vi "Data_get.vi"() -> ()   [LabVIEW 2009]
uses:
  <vilib>/Analysis/2dsp.llb/Real FFT.vi
  <vilib>/Analysis/NI_AALPro.lvlib
panel:
  in  "Repetition rate (Hz)":ext=2.5
  in  "Chirp start (MHz)":ext=2.5
  in  "Filter up to (MHz)":ext=2.5
  in  "Amount of averagings":u32
  out "Data":dbl[](array[numeric])
  out "XY Graph 5":cluster{ext[], dbl[]}(graph)
  out "FFT (Im)":dbl[](array[numeric])
  out "FFT (Re)":dbl[](array[numeric])
  out "Final array":ext[][](array[numeric])
  out "size(s)":i32
  in  "ns/div":u32
  in  "ps/point":u32
  out "Oscilloscope Data":dbl[](array[numeric])
  in  "Channel Number":u16=1
  out "Oscilloscope graph":dbl[](graph)
  in  "Stop":bool
  in  "TDS VISA Port":refnum<visa-resource-name>="GPIB0::1::INSTR"
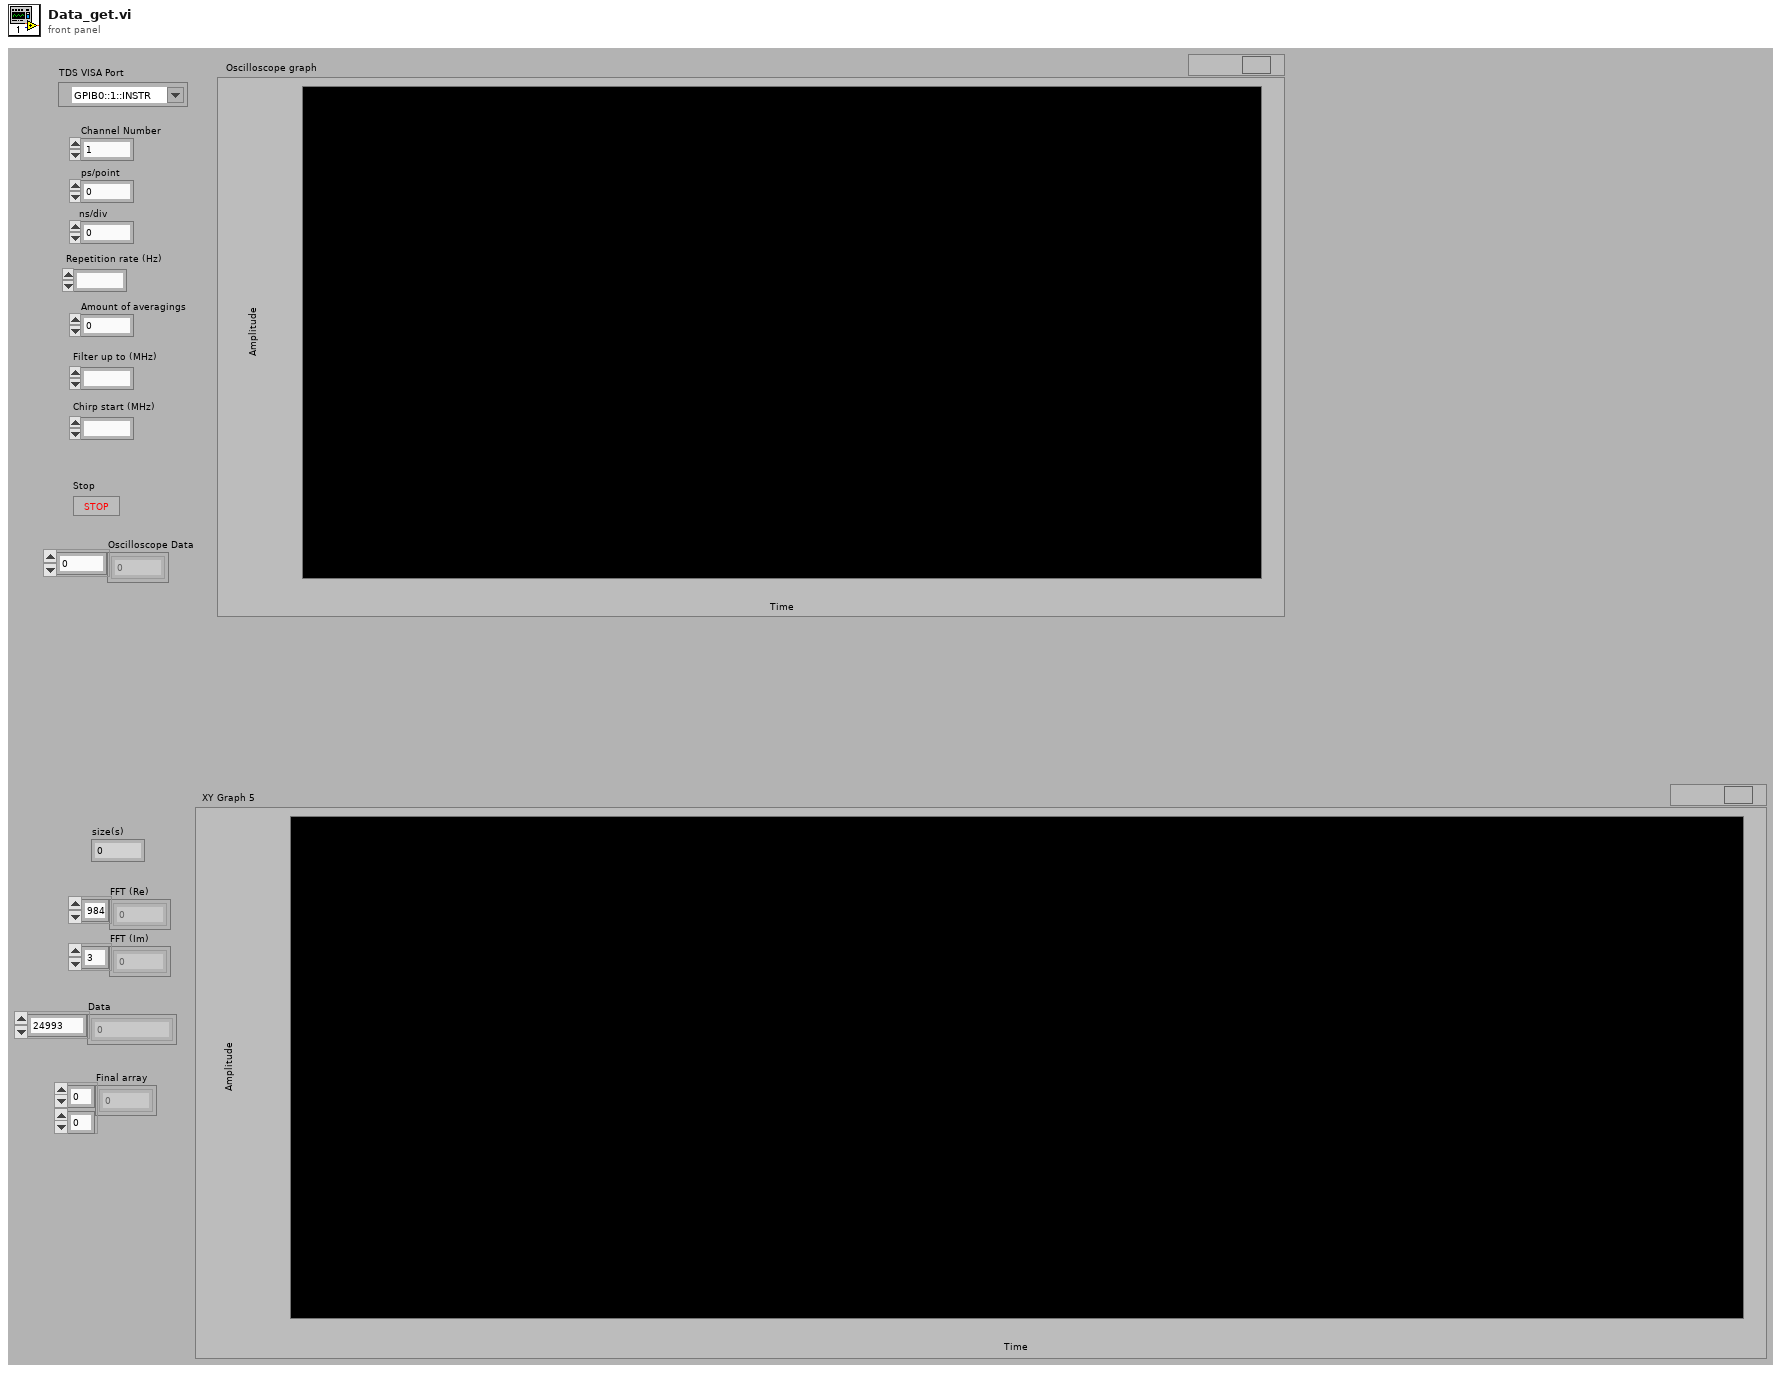
[diagram p1: front panel]
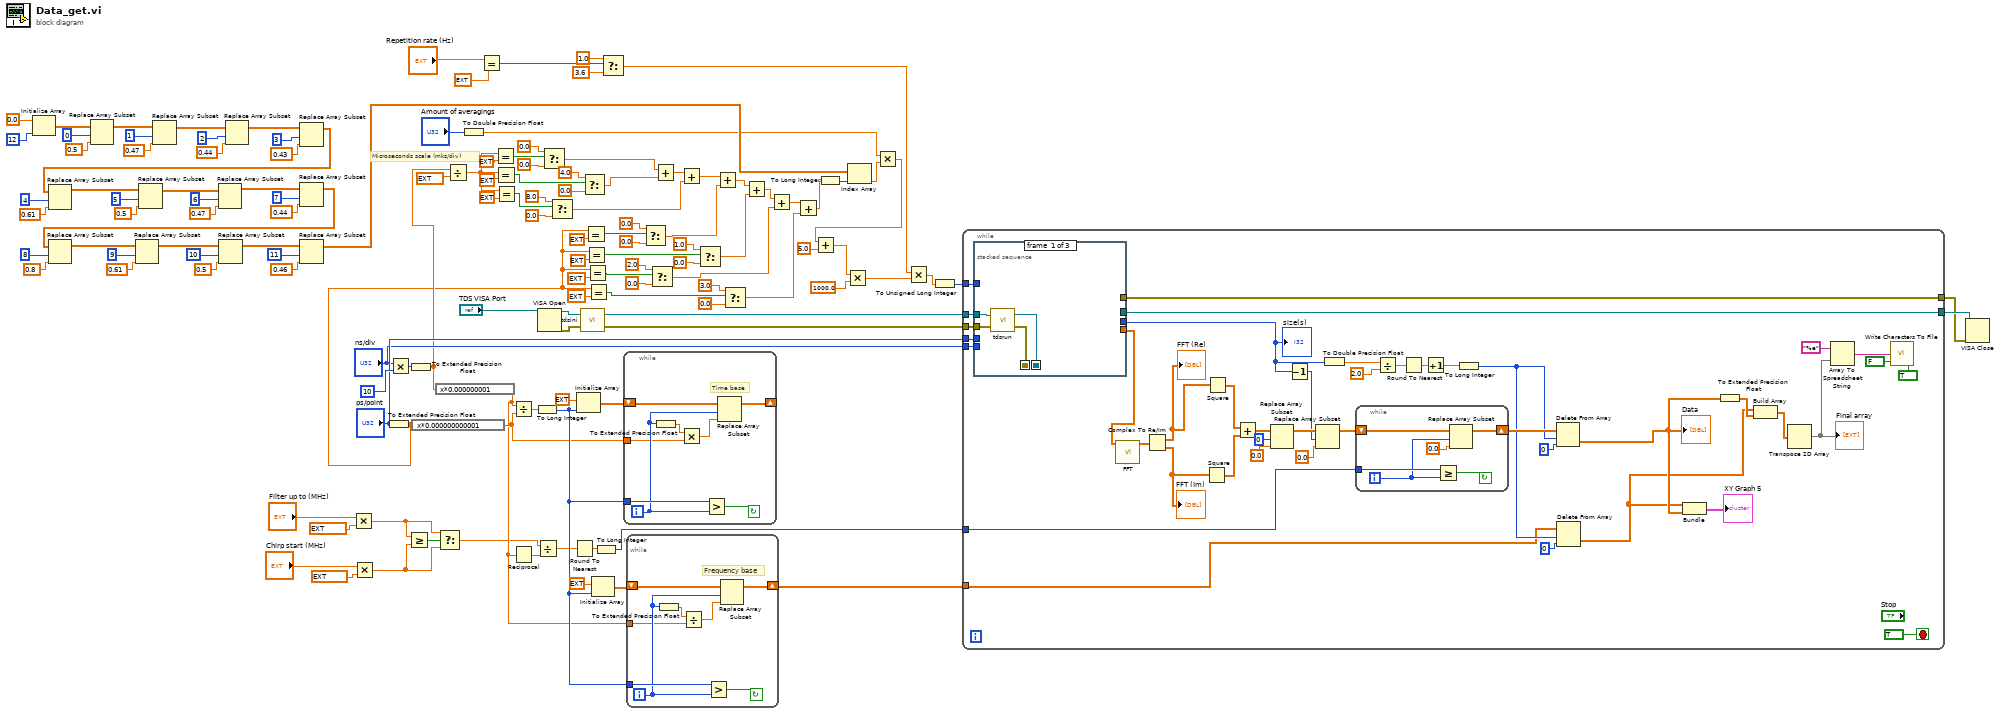
[diagram p0: block diagram]
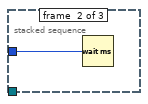
[diagram p2: hidden frame]
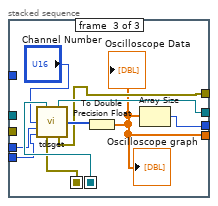
[diagram p3: hidden frame]
diagram:
  # "Microseconds scale (mks/div)"
  n1 = Initialize Array(0.0 ("element"), 12 ("dimension size")) -> (w109:dbl[])
  n2 = Replace Array Subset(array=w109, new element=0.5 ("new element/subarray"), index=0) -> (w104:dbl[])
  n3 = Replace Array Subset(array=w104, new element=0.47 ("new element/subarray"), index=1) -> (w83:dbl[])
  n4 = Replace Array Subset(array=w83, new element=0.44 ("new element/subarray"), index=2) -> (w82:dbl[])
  n5 = Replace Array Subset(array=w82, new element=0.43 ("new element/subarray"), index=3) -> (w81:dbl[])
  n6 = Replace Array Subset(array=w81, new element=0.61 ("new element/subarray"), index=4) -> (w80:dbl[])
  n7 = Replace Array Subset(array=w80, new element=0.5 ("new element/subarray"), index=5) -> (w79:dbl[])
  n8 = Replace Array Subset(array=w79, new element=0.47 ("new element/subarray"), index=6) -> (w78:dbl[])
  n9 = Replace Array Subset(array=w78, new element=0.44 ("new element/subarray"), index=7) -> (w77:dbl[])
  n10 = Replace Array Subset(array=w77, new element=0.8 ("new element/subarray"), index=8) -> (w76:dbl[])
  n11 = Replace Array Subset(array=w76, new element=0.61 ("new element/subarray"), index=9) -> (w75:dbl[])
  n12 = Replace Array Subset(array=w75, new element=0.5 ("new element/subarray"), index=10) -> (w74:dbl[])
  n13 = Replace Array Subset(array=w74, new element=0.46 ("new element/subarray"), index=11) -> (w32:dbl[])
  n14 = Multiply(x="Filter up to (MHz)", y=ext 1000000.0) -> (x*y=w12:ext)
  n15 = Multiply(x="Chirp start (MHz)", y=ext 1000000.0) -> (x*y=w9:ext)
  n16 = To Extended Precision Float(1:"ps/point") -> (0:w25:ext)
  n17 = Multiply(x="ns/div", y=u32 10) -> (x*y=w125:u32)
  n18 = Greater Or Equal?(x=w12, y=w9) -> (x >= y?=w21:bool)
  n19 = To Extended Precision Float(1:w125) -> (0:w113:ext)
  n20 = expression code="x*0.000000000001"(w25) -> (w114:ext)
  n21 = expression code="x*0.000000001"(w113) -> (w20:ext)
  n22 = Select(t=w12, s=w21, f=w9) -> (s? t:f=w18:ext)
  n23 = Divide(x=w113, y=ext 10000.0) -> (x/y=w73:ext)
  n24 = To Double Precision Float(number="Amount of averagings") -> (double precision float=w28:dbl)
  n25 = Equal?(x="Repetition rate (Hz)", y=ext 2.5) -> (x = y?=w7:bool)
  n26 = Equal?(x=w73, y=ext 1.0) -> (x = y?=w65:bool)
  n27 = Equal?(x=w73, y=ext 2.0) -> (x = y?=w60:bool)
  n28 = Equal?(x=w73, y=ext 4.0) -> (x = y?=w57:bool)
  n29 = Divide(x=w20, y=w114) -> (x/y=w124:ext)
  n30 = Reciprocal(x=w20) -> (1/x=w19:ext)
  n31 = To Long Integer(number=w124) -> (32bit integer=w116:i32)
  n32 = Divide(x=w18, y=w19) -> (x/y=w17:ext)
  n33 = VISA Open(VISA resource name="TDS VISA Port") -> (VISA resource name=w130:refnum<visa-resource-name>, error out=w131:errorcluster)  [unwired: 4 in]
  n34 = Select(t=0.0, s=w65, f=0.0) -> (s? t:f=w44:dbl)
  n35 = Select(t=8.0, s=w57, f=0.0) -> (s? t:f=w41:dbl)
  n36 = Round To Nearest(number=w17) -> (nearest integer value=w16:ext)
  n37 = Initialize Array(ext 0.0 ("element"), w116) -> (w120:ext[])
  n38 = call "tdsini.vi"("Error In (No Error)"=w131, "VISA Port In"=w130) -> ("Error Out"=w132:errorcluster, "VISA Port Out"=w133:refnum<visa-resource-name>)
  n39 = Select(t=4.0, s=w60, f=0.0) -> (s? t:f=w43:dbl)
  n40 = Equal?(x=w25, y=ext 25.0) -> (x = y?=w48:bool)
  n41 = Equal?(x=w25, y=ext 50.0) -> (x = y?=w47:bool)
  n42 = Equal?(x=w25, y=ext 100.0) -> (x = y?=w46:bool)
  n43 = Equal?(x=w25, y=ext 200.0) -> (x = y?=w45:bool)
  n44 = Initialize Array(ext 0.0 ("element"), w116) -> (w118:ext[])
  n45 = To Long Integer(number=w16) -> (32bit integer=w15:i32)
  n46 = Select(t=1.0, s=w7, f=3.6) -> (s? t:f=w4:dbl)
  n47 = while {
    tunnel: w116 -> [w140]
    shift-right: [w138] -> _
    shift-left: w120 -> [w139]
    tunnel: w114 -> [w135]
    i -> [w137]
    stop <- w141 continue-if-true
    # "Time base"
    n48 = To Extended Precision Float(1:w137) -> (0:w136:ext)
    n49 = Multiply(x=w136, y=w135) -> (x*y=w134:ext)
    n50 = Greater?(x=w140, y=w137) -> (0:w141:bool)
    n51 = Replace Array Subset(array=w139, new element=w134, index=w137) -> (w138:ext[])
  }
  n52 = while {
    tunnel: w116 -> [w148]
    shift-right: [w146] -> w117
    shift-left: w118 -> [w147]
    tunnel: w20 -> [w143]
    i -> [w145]
    stop <- w149 continue-if-true
    # "Frequency base"
    n53 = To Extended Precision Float(1:w145) -> (0:w144:ext)
    n54 = Divide(x=w144, y=w143) -> (x/y=w142:ext)
    n55 = Greater?(x=w148, y=w145) -> (0:w149:bool)
    n56 = Replace Array Subset(array=w147, new element=w142, index=w145) -> (w146:ext[])
  }
  n57 = Select(t=0.0, s=w48, f=0.0) -> (s? t:f=w39:dbl)
  n58 = Select(t=2.0, s=w46, f=0.0) -> (s? t:f=w35:dbl)
  n59 = Add(x=w44, y=w43) -> (x+y=w42:dbl)
  n60 = Add(x=w42, y=w41) -> (x+y=w40:dbl)
  n61 = Select(t=1.0, s=w47, f=0.0) -> (s? t:f=w37:dbl)
  n62 = Add(x=w40, y=w39) -> (x+y=w38:dbl)
  n63 = Select(t=3.0, s=w45, f=0.0) -> (s? t:f=w33:dbl)
  n64 = Add(x=w38, y=w37) -> (x+y=w36:dbl)
  n65 = Add(x=w36, y=w35) -> (x+y=w34:dbl)
  n66 = Add(x=w34, y=w33) -> (x+y=w30:dbl)
  n67 = To Long Integer(number=w30) -> (32bit integer=w31:i32)
  n68 = Index Array(array=w32, index=w31) -> (element=w29:dbl)
  n69 = Multiply(x=w28, y=w29) -> (x*y=w24:dbl)
  n70 = Add(x=w24, y=5.0) -> (x+y=w22:dbl)
  n71 = Multiply(x=w22, y=1000.0) -> (x*y=w3:dbl)
  n72 = Multiply(x=w4, y=w3) -> (x*y=w2:dbl)
  n73 = To Unsigned Long Integer(number=w2) -> (unsigned 32bit integer=w26:u32)
  n74 = while {
    tunnel: [w189] -> w127
    tunnel: [w190] -> w128
    tunnel: w132 -> [w191]
    tunnel: w133 -> [w192]
    tunnel: "ps/point" -> [w188]
    tunnel: "ns/div" -> [w187]
    tunnel: w117 -> [w151]
    tunnel: w26 -> [w168]
    tunnel: w15 -> [w164]
    stop <- TRUE stop-if-true
    n75 = stacked-sequence {
      seq-local: [w200 _ _] -> [_ _ w213]
      seq-local: [w199 _ _] -> [_ _ w206]
      tunnel: w192 -> [w201 _ _]
      tunnel: w191 -> [w202 _ _]
      tunnel: [_ _ w211] -> w190
      tunnel: [_ _ w210] -> w189
      tunnel: w188 -> [_ _ w208]
      tunnel: w187 -> [_ _ w207]
      tunnel: [_ _ w205] -> w162
      tunnel: [_ _ w204] -> w180
      tunnel: w168 -> [_ w203 _]
      frame #0 {
        n76 = call "tdsrun.vi"("Error In (No Error)"=w202, "VISA Port In"=w201) -> ("Error Out"=w199:errorcluster, "VISA Port Out"=w200:refnum<visa-resource-name>)
      }
      frame #1 {
        n77 = Wait (ms)(milliseconds to wait=w203) -> ()  [unwired: 1 out]
      }
      frame #2 {
        n78 = call "tdsget.vi"("VISA Port In"=w213, "Channel Number"="Channel Number", "ps/point"=w208, "ns/div"=w207, "Error In (No Error)"=w206) -> ("VISA Port Out"=w211:refnum<visa-resource-name>, "TDS Data"=w212:u16[], "Error Out"=w210:errorcluster)  [unwired: 8 in]
        n79 = To Double Precision Float(number=w212) -> (double precision float=w204:dbl[])
        "Oscilloscope graph" <- w204
        "Oscilloscope Data" <- w204
        n80 = Array Size(array=w204) -> (size(s)=w205:i32)
      }
    }
    "size(s)" <- w162
    n81 = call-poly <vilib>:"FFT.vi"("X"=w180) -> ("FFT {X}"=w186:cdb[])  [unwired: 9 in, 1 out]
    n82 = Complex To Re/Im(x + iy=w186) -> (x=w185:dbl[], y=w184:dbl[])
    "FFT (Re)" <- w185
    "FFT (Im)" <- w184
    n83 = Square(x=w184) -> (x^2=w182:dbl[])
    n84 = Square(x=w185) -> (x^2=w183:dbl[])
    n85 = Add(x=w183, y=w182) -> (x+y=w172:dbl[])
    n86 = Replace Array Subset(array=w172, new element=0.0 ("new element/subarray"), index=0) -> (w171:dbl[])
    n87 = Decrement(x=w162) -> (x-1=w170:i32)
    n88 = Replace Array Subset(array=w171, new element=0.0 ("new element/subarray"), index=w170) -> (w165:dbl[])
    n89 = To Double Precision Float(number=w162) -> (double precision float=w161:dbl)
    n90 = while {
      tunnel: w164 -> [w197]
      shift-right: [w195] -> w163
      shift-left: w165 -> [w196]
      i -> [w194]
      stop <- w198 continue-if-true
      n91 = Greater Or Equal?(x=w197, y=w194) -> (x >= y?=w198:bool)
      n92 = Replace Array Subset(array=w196, new element=0.0 ("new element/subarray"), index=w194) -> (w195:dbl[])
    }
    n93 = Divide(x=w161, y=2.0) -> (x/y=w159:dbl)
    n94 = Round To Nearest(number=w159) -> (nearest integer value=w158:dbl)
    n95 = Increment(x=w158) -> (x+1=w157:dbl)
    n96 = To Long Integer(number=w157) -> (32bit integer=w152:i32)
    n97 = Delete From Array(array=w163, length=w152, index=0) -> (deleted portion=w155:dbl[])  [unwired: 1 out]
    "Data" <- w155
    n98 = Delete From Array(array=w151, length=w152, index=0) -> (deleted portion=w150:ext[])  [unwired: 1 out]
    n99 = Bundle(w150, w155) -> (→"XY Graph 5":cluster{ext[], dbl[]})  [unwired: 1 in]
    n100 = To Extended Precision Float(1:w155) -> (0:w154:ext[])
    n101 = Build Array(w150, w154) -> (w166:ext[][])
    n102 = Transpose 2D Array(2D array=w166) -> (transposed array=w178:ext[][])
    "Final array" <- w178
    n103 = Array To Spreadsheet String(array=w178, 3:"%e") -> (spreadsheet string=w175:string)  [unwired: 1 in]
    n104 = call <vilib>:"Write Characters To File.vi"("convert eol? (no:F)"=TRUE, "append to file? (new file:F)"=FALSE, "character string"=w175) -> ()  [unwired: 2 in, 1 out]
  }
  n105 = VISA Close(VISA resource name=w128, error in (no error)=w127) -> ()  [unwired: 1 out]
